vi "Write Return VF Device UID Msg.vi"(10 "Return VF Device UID Msg":refnum<class "Return VF Device UID Msg.lvclass">, 11 "Optimization in":refnum<class "Optimization.lvclass">) -> (3 "Optimization out":refnum<class "Optimization.lvclass">)   [LabVIEW 2016, in "Optimization Framework.lvlib" / "Optimization.lvclass"]
uses:
  Optimization.lvclass
  Optimization Messages/Return VF Device UID Msg/Return VF Device UID Msg.lvclass
  Optimization.lvclass/Optimization.ctl
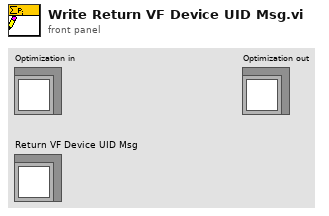
[diagram p1: front panel]
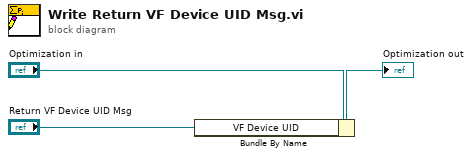
[diagram p0: block diagram]
diagram:
  n1 = Bundle By Name(cluster="Optimization in", "VF Device UID"="Return VF Device UID Msg") -> (→"Optimization out":refnum<class "Optimization.lvclass">)
